vi "Write Number of Channels.vi"(8 "error in (no error)":errorcluster, 10 "Number of Channels":i32, 11 "Mag Lab Digitizer in":refnum<class "Mag Lab Digitizer.lvclass">) -> (0 "error out":errorcluster, 3 "Mag Lab Digitizer out":refnum<class "Mag Lab Digitizer.lvclass">)   [LabVIEW 2015, in "Mag Lab Digitizer.lvclass"]
uses:
  Mag Lab Digitizer.lvclass
  Mag Lab Digitizer.lvclass/Mag Lab Digitizer.ctl
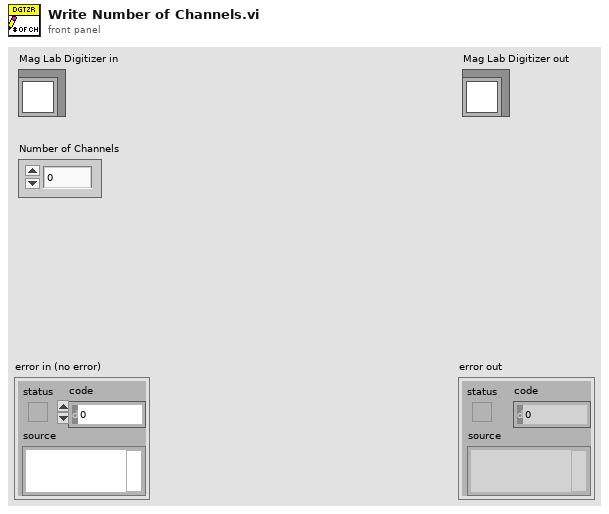
[diagram p1: front panel]
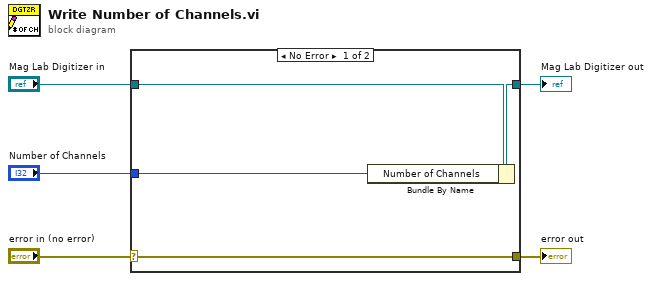
[diagram p0: block diagram]
diagram:
  n1 = case shown="No Error" "error in (no error)" {
    selector: "error in (no error)" -> [w9 w10]
    tunnel: [w9 w10] -> w4
    tunnel: [w7 w11] -> w2
    tunnel: "Mag Lab Digitizer in" -> [w8 w11]
    tunnel: "Number of Channels" -> [w6 _]
    frame No Error {
      n2 = Bundle By Name(cluster=w8, "Number of Channels"=w6) -> (w7:refnum<class "Mag Lab Digitizer.lvclass">)
    }
    frame Error {
    }
  }
  "error out" <- w4
  "Mag Lab Digitizer out" <- w2
